vi "After.vi"(7 "Actor in":refnum<class "Actor.lvclass">, 8 "Error in":errorcluster, 10 "Msg DVR in":refnum<data-value>) -> (0 "Error out":errorcluster, 2 "Msg DVR out":refnum<data-value>, 5 "Actor out":refnum<class "Actor.lvclass">)   [LabVIEW 2020, in "_Template.lvlib" / "Templates.lvlib" / "TEMPLATE jettl Msg.lvlib" / "TEMPLATE Msg Contents.lvclass"]
uses:
  TEMPLATE Msg Contents.lvclass
  TEMPLATE Msg Contents.lvclass/TEMPLATE Msg Contents.ctl
  TEMPLATE jettl Msg/TEMPLATE jettl Msg.lvclass
  jettl/jettl/Actor/Actor.lvclass
  jettl/jettl/Unified Actor Relation.ctl
  jettl/jettl/jettl.lvlib
  jettl/jettl/Teller.ctl
  jettl/jettl/Msg Contents/Msg Contents.lvclass
  jettl/jettl/Msg.ctl
  jettl/jettl/Msg/Msg.lvclass
panel:
  # "This front panel should not be manipulated."
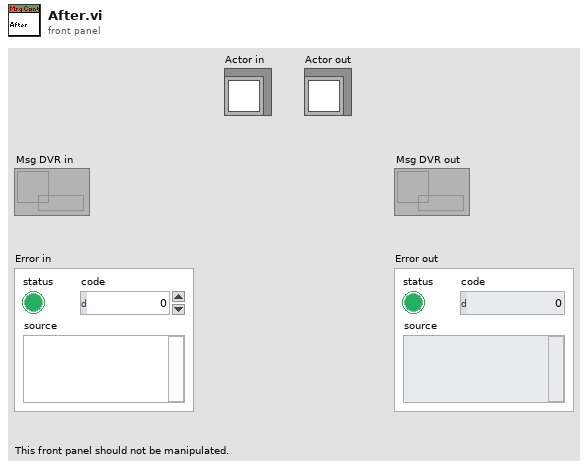
[diagram p1: front panel]
types:
  T1 = typedef "jettl.lvlib/Msg.ctl" = cluster{"Msg":refnum<class "Msg.lvclass">, "Msg Contents":refnum<class "Msg Contents.lvclass">, "Teller":T2}
  T2 = typedef "jettl.lvlib/Teller.ctl" = cluster{"Unified Actor Alias":string, "Unified Actor Relation":T3, "Absolute Time":timestamp, "Relative Time":dbl}
  T3 = typedef "jettl.lvlib/Unified Actor Relation.ctl" = enum16{"Self", "Parent", "Child"}
  T4 = typedef "_Template.lvlib/Templates.lvlib/TEMPLATE jettl Msg.lvlib/Data.ctl" = cluster{"Placeholder Data":bool}
  T5 = typedef "_Template.lvlib/Templates.lvlib/TEMPLATE jettl Msg.lvlib/Metadata.ctl" = cluster{"Placeholder Metadata":bool}
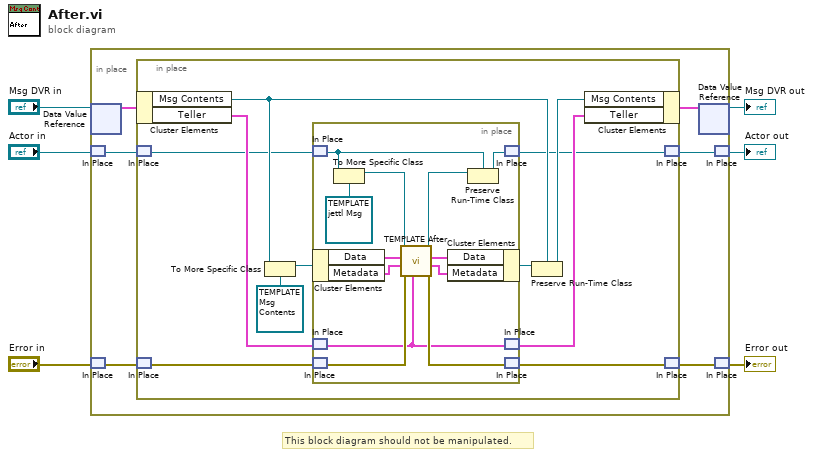
[diagram p0: block diagram]
diagram:
  # "This block diagram should not be manipulated."
  n1 = in-place {
    n2 = in-place-dvr #1("Msg DVR in") -> (w11:T1)  [unwired: 1 out]
    n3 = in-place-match #2("Actor in") -> (w8:refnum<class "Actor.lvclass">)
    n4 = in-place-match #3("Error in") -> (w10:errorcluster)
    n5 = in-place {
      n6 = in-place-cluster #4(w11) -> ("Msg Contents"=w22:refnum<class "Msg Contents.lvclass">, "Teller"=w16:T2)
      n7 = in-place-match #5(w8) -> (w14:refnum<class "Actor.lvclass">)
      n8 = in-place-match #6(w10) -> (w18:errorcluster)
      n9 = To More Specific Class(target class=refnum<class "TEMPLATE Msg Contents.lvclass"> refnum ("_Template.lvlib:Templates.lvlib:TEMPLATE jettl Msg.lvlib:TEMPLATE Msg Contents.lvclass"), reference=w22) -> (specific class reference=w23:refnum<class "TEMPLATE Msg Contents.lvclass">)  [unwired: 1 in, 1 out]
      n10 = in-place {
        n11 = in-place-match #7(w14) -> (w25:refnum<class "Actor.lvclass">)
        n12 = in-place-cluster #8(w23) -> ("Data"=w34:T4, "Metadata"=w30:T5)
        n13 = in-place-match #9(w16) -> (w24:T2)
        n14 = in-place-match #10(w18) -> (w28:errorcluster)
        n15 = To More Specific Class(target class=refnum<class "TEMPLATE jettl Msg.lvclass"> refnum ("_Template.lvlib:Templates.lvlib:TEMPLATE jettl Msg.lvlib:TEMPLATE jettl Msg.lvclass"), reference=w25) -> (specific class reference=w32:refnum<class "TEMPLATE jettl Msg.lvclass">)  [unwired: 1 in, 1 out]
        n16 = call-dynamic "TEMPLATE After.vi"("Teller"=w24, "Error in"=w28, "Metadata in"=w30, "Data in"=w34, "TEMPLATE jettl Msg in"=w32) -> ("Error out"=w27:errorcluster, "Metadata out"=w29:T5, "Data out"=w33:T4, "TEMPLATE jettl Msg out"=w31:refnum<class "TEMPLATE jettl Msg.lvclass">)  [unwired: 3 in]
        n17 = in-place-cluster #8("Data"=w33, "Metadata"=w29) -> (w21:refnum<class "TEMPLATE Msg Contents.lvclass">)
        n18 = Preserve Run-Time Class(object in=w31, 2:w25) -> (object out=w26:refnum<class "Actor.lvclass">)  [unwired: 1 in, 1 out]
        n19 = in-place-match #7(w26) -> (w13:refnum<class "Actor.lvclass">)
        n20 = in-place-match #9(w24) -> (w15:T2)
        n21 = in-place-match #10(w27) -> (w17:errorcluster)
      }
      n22 = Preserve Run-Time Class(object in=w21, 2:w22) -> (object out=w20:refnum<class "Msg Contents.lvclass">)  [unwired: 1 in, 1 out]
      n23 = in-place-cluster #4("Msg Contents"=w20, "Teller"=w15) -> (w12:T1)
      n24 = in-place-match #5(w13) -> (w7:refnum<class "Actor.lvclass">)
      n25 = in-place-match #6(w17) -> (w9:errorcluster)
    }
    n26 = in-place-dvr #1(w12) -> (→"Msg DVR out":refnum<data-value>)  [unwired: 1 out]
    n27 = in-place-match #2(w7) -> (→"Actor out":refnum<class "Actor.lvclass">)
    n28 = in-place-match #3(w9) -> (→"Error out":errorcluster)
  }
